vi "Step 1 - Design Lowpass (Lowpass).vi"() -> ()   [LabVIEW 2023]
doc: "Demonstrates how to use the Classical Filter Design Express VI to design a lowpass finite impulse response (FIR) filter and how to use the Filter Analysis Express VI to analyze the characteristics of the designed filter.\n\nComplete the following steps to use this VI.\n1) Open the block diagram of the VI.\n2) Double-click the Equi-Ripple FIR Lowpass Filter Express VI to open the configuration dialog box of the Classical Filter Design Express VI.\n<B>Note:</B> The original name of the Express VI is Classical Filter Design. After you enter specifications in the configuration dialog box and click the <B>OK</B> button, the name of the Express VI on the block diagram changes to reflect the type of filter you design. In this example, the name changes to Equi-Ripple FIR Lowpass Filter.\n3) Set the <B>Sampling frequency</B> to 10000.\n4) Set the <B>Passband edge frequency</B> to 100.\n5) Remove the checkmark from the <B>Magnitude in dB</B> checkbox and set the <B>Passband ripple</B> to 0.0025.\n6) Set the <B>Stopband edge frequency</B> to 800.\n7) Place a checkmark in the <B>Magnitude in dB</B> checkbox and set the <B>Stopband attenuation</B> to 60.\n8) Set the <B>Design method</B> to Equi-Ripple FIR.\n9) Observe the magnitude response and filter order on the <B>Configure Classical Filter Design</B> dialog box.\n10) Click the <B>OK</B> button.\n11) Run the VI.\n12) Observe the magnitude response of the designed filter on the front panel."
panel:
  out "Magnitude Response":dynamicdata(graph) caption="magnitude"
  # "Select Help>>Show Context Help and move the cursor over the VI icon for more information."
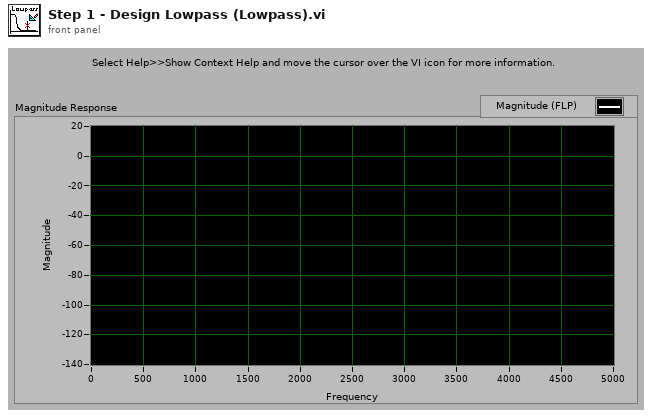
[diagram p1: front panel]
types:
  T1 = typedef "NI_DigFilterLicensed.lvlib/DFD Filter Obj.ctl" = cluster{"mSRate_Fs":dbl, "mSRate_Version":string, "mSRate_Comments":string, "mSRate_OrgCoef":T2, "mSRate_CurCoef":T2, "mSRate_Quantized?":bool, "mSRate_QCoef":T2, "mSRate_QSettings":T4[], "mSRate_Order":i32, "mSRate_Scaling":cluster{"mSRate_ScaleByPowerOf2?":bool, "mSRate_ScaleType":T6}}
  T2 = typedef "NI_DigFilterLicensed.lvlib/DFD Filter Coef.ctl" = cluster{"type":T3, "gain":dbl, "coef a (k)":dbl[], "coef b (v)":dbl[]}
  T3 = typedef "NI_DigFilterLicensed.lvlib/DFD Filter Structure Type Selector.ctl" = enum16{"Undefined", "FIR Direct Form", "FIR Direct Form Transposed", "FIR Symmetric", "FIR Antisymmetric", "IIR Direct Form I", "IIR Direct Form I Transposed", "IIR Direct Form II", "IIR Direct Form II Transposed", "IIR Cascaded Second Order Sections Form I", "IIR Cascaded Second Order Sections Form I Transposed", "IIR Cascaded Second Order Sections Form II", "IIR Cascaded Second Order Sections Form II Transposed", "Lattice Allpass (basic sections)", "Lattice Allpass (one multiplier sections)", "Lattice Allpass (normalized sections)", "Lattice AR (basic sections)", "Lattice AR (one multiplier sections)", "Lattice AR (normalized sections)", "Lattice MA (minimum phase)", "Lattice MA (maximum phase)", "Lattice ARMA (basic sections)", "Lattice ARMA (one multiplier sections)", "Lattice ARMA (normalized sections)"}
  T4 = typedef "NI_DigFilterLicensed.lvlib/dfd_Internal Quantization Settings.ctl" = cluster{"source":T5, "wl":i16, "iwl":i16, "overflow mode":enum16{"Saturation", "Wrap"}, "rounding mode":enum16{"Nearest", "Truncation"}, "signed?":bool}
  T5 = typedef "NI_DigFilterLicensed.lvlib/dfd_Internal Quantization Srcs.ctl" = u16
  T6 = typedef "NI_DigFilterLicensed.lvlib/DFD Coef Norm Type.ctl" = enum16{"No Norm", "Time Domain 1-Norm", "Time Domain 2-Norm", "Time Domain Inf-Norm"}
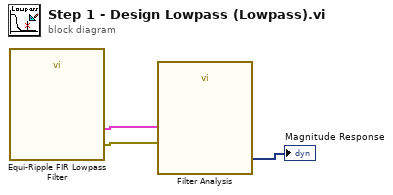
[diagram p0: block diagram]
diagram:
  n1 = call "Equi-Ripple FIR Lowpass Filter"() -> ("error out"=w2:errorcluster, "filter out"=w3:T1)  [unwired: 1 in, 9 out]
  n2 = call "Filter Analysis"("error in (no error)"=w2, "filter in"=w3) -> ("magnitude"=→"Magnitude Response":dynamicdata)  [unwired: 9 out]
